vi "Read Remote IP Address.vi"(11 "TCP Stream in":refnum<class "TCP Stream.lvclass">) -> (2 "Remote IP":string)   [LabVIEW 2020, in "TCP Stream.lvclass"]
doc: "Returns the IP address of the remote connection."
uses:
  TCP Stream.lvclass
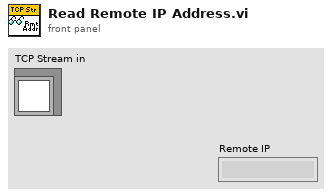
[diagram p1: front panel]
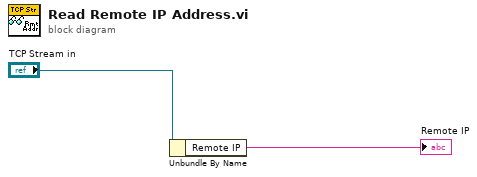
[diagram p0: block diagram]
diagram:
  n1 = Unbundle By Name("TCP Stream in") -> ("Remote IP"=→"Remote IP":string)
